vi "Trim All Spaces.vi"(8 "error in (no error)":errorcluster, 11 "Label.Text":string) -> (0 "error out":errorcluster, 3 "result string":string)   [LabVIEW 2018]
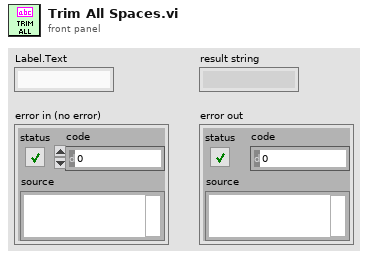
[diagram p1: front panel]
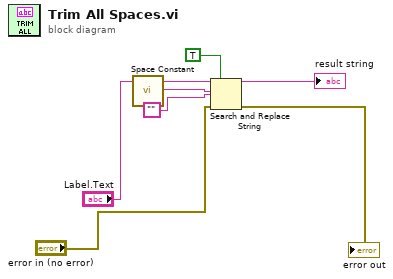
[diagram p0: block diagram]
diagram:
  n1 = call <vilib>:"Space Constant.vi"() -> ("String"=w2:string)
  n2 = Search and Replace String(replace all?=TRUE ("replace all? (F)"), input string="Label.Text", search string=w2, replace string="", error in="error in (no error)") -> (result string=→"result string":string, error out=→"error out":errorcluster)  [unwired: 3 in, 2 out]
